vi "Periodic Tasks.vi"(8 "error in":errorcluster) -> ()   [LabVIEW 2013]
doc: "This VI runs in parallel to other tasks. It can contain as many user-defined periodic loops as you need. These can carry out PID or other sorts of timed response."
uses:
  <vilib>/Rock Robotics/WPI/Solenoid/WPI_SolenoidValue.ctl
  Drive State.ctl
  <vilib>/Rock Robotics/SystemInterfaces/Utilities/FPGA_UtilitiesLED Source.ctl
  <vilib>/Rock Robotics/SystemInterfaces/Utilities/FPGA_UtilitiesLED State.ctl
  Robot Global Data.vi
  <vilib>/Rock Robotics/WPI/Solenoid/Deprecated/WPI_SolenoidGetBool.vi
  <vilib>/Rock Robotics/WPI/Solenoid/WPI_SolenoidSetEnum.vi
  <vilib>/addons/control/pid/pid.llb/PID (DBL).vi
  <vilib>/addons/control/pid/NI_PID_pid.lvlib
panel:
  in  "Shot Time":u32
  in  "ANGLE PID":T1={"proportional gain (Kc)"=0.01, "integral time (Ti, min)"=0.0, "derivative time (Td, min)"=0.0}
  in  "Shooter Power 2":dbl=1.0
  out "Conveyor Out":dbl
  out "BM Output":dbl
  out "Arm Out":T2
  in  "Low Power":dbl=0.15
  in  "High Power":dbl=1.0
  in  "Arm Down Cov Power":dbl=0.4 format="%#_13g"
  in  "Center Power":dbl=0.2
  in  "Yaw Rate x Constant":dbl=0.1 format="%#_13g"
  in  "Rot Threshold":dbl=0.08 format="%#_13g"
  in  "FL PID":T1={"proportional gain (Kc)"=0.01, "integral time (Ti, min)"=0.1, "derivative time (Td, min)"=0.0}
  in  "FR PID":T1={"proportional gain (Kc)"=0.01, "integral time (Ti, min)"=0.1, "derivative time (Td, min)"=0.0}
  in  "BL PID":T1={"proportional gain (Kc)"=0.01, "integral time (Ti, min)"=0.1, "derivative time (Td, min)"=0.0}
  in  "BR PID":T1={"proportional gain (Kc)"=0.01, "integral time (Ti, min)"=0.1, "derivative time (Td, min)"=0.0}
  out "ANGULAR\nRATE":dbl(knob) scale=-100.0..100.0
  out "ANGLE":dbl(slide) scale=-180.0..180.0
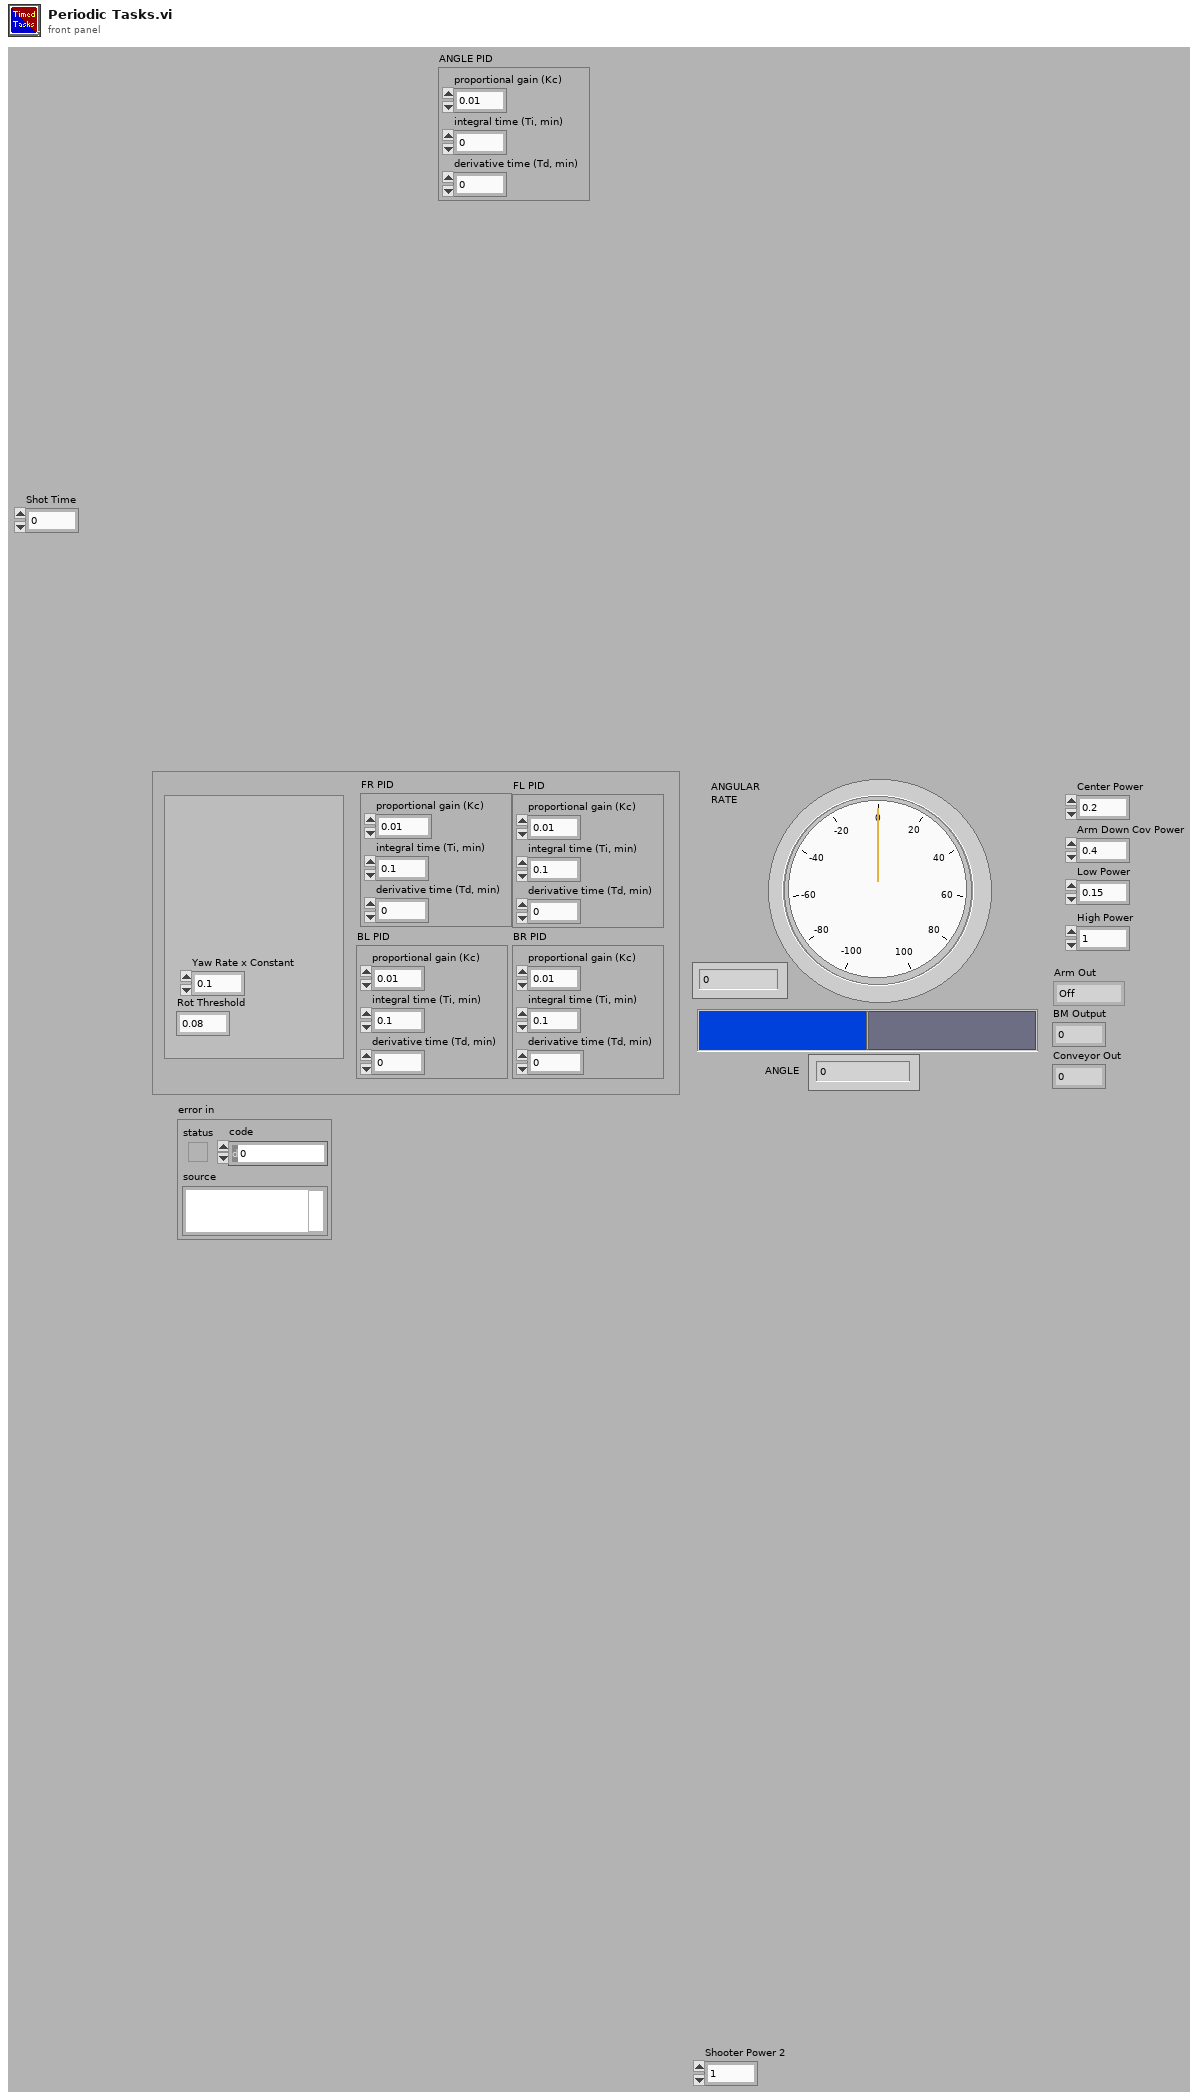
[diagram p1: front panel]
types:
  T1 = cluster{"proportional gain (Kc)":dbl, "integral time (Ti, min)":dbl, "derivative time (Td, min)":dbl}
  T2 = typedef "WPI_SolenoidValue.ctl" = enum16{"Off", "On", "Forward", "Reverse"}
  T3 = typedef "Drive State.ctl" = enum16{"Knob Control", "Straight PID", "Reset Mode"}
  T4 = typedef "WPI_MotorControlDeviceRef.ctl" = cluster{"DeviceStatus":errorcluster, "Type":enum16{"PWM", "CAN"}, "PWM":cluster{"Digital Module":T5, "PWM Channel":T6, "DeadBand":T7}, "CAN":cluster{"Device Number":u8, "Control Mode":T8, "Semaphore":T9, "Max Vout":dbl}, "Invert":bool, "TransformRef":T10, "InvTransformRef":T10}
  T5 = typedef "FPGA_TypedefDigitalModule.ctl" = enum16{"Digital Module 1", "Digital Module 2"}
  T6 = typedef "FPGA_DIOPWMChannel.ctl" = enum8{"PWM 1", "PWM 2", "PWM 3", "PWM 4", "PWM 5", "PWM 6", "PWM 7", "PWM 8", "PWM 9", "PWM 10", "Invalid"}
  T7 = typedef "WPI_PWMDeadband.ctl" = cluster{"Name":string, "maxPositivePwm":i32, "minPositivePwm":i32, "centerPwm":i32, "maxNegativePwm":i32, "minNegativePwm":i32, "angularRange":u16}
  T8 = typedef "WPI_CANJaguar_ControlMode.ctl" = enum8{"Percent VBus", "Current", "Speed", "Position", "Voltage"}
  T9 = typedef "Semaphore RefNum" = refnum<k1>
  T10 = typedef "WPI_PWMTransform_ConPane.ctl" = refnum<vi>
  T11 = typedef "WPI_EncoderDevRef.ctl" = cluster{"DevStatus":errorcluster, "EncoderIndex":T12, "CounterIndex":T13, "DistancePerCount":dbl, "Decoding Type":T14}
  T12 = typedef "FPGA_EncoderIdx.ctl" = enum8{"Enc 0", "Enc 1", "Enc 2", "Enc 3", "Invalid"}
  T13 = typedef "FPGA_CounterCtrSystemIndex.ctl" = enum8{"Ctr 0", "Ctr 1", "Ctr 2", "Ctr 3", "Ctr 4", "Ctr 5", "Ctr 6", "Ctr 7", "Invalid"}
  T14 = typedef "WPI_EncoderType.ctl" = enum16{"1x", "2x", "4x"}
  T15 = typedef "WPI_DigitalInputDevRef.ctl" = cluster{"DevStatus":errorcluster, "DIO Channel":T16, "Digital Module":T5}
  T16 = typedef "FPGA_DIOChannel.ctl" = enum8{"DIO 1", "DIO 2", "DIO 3", "DIO 4", "DIO 5", "DIO 6", "DIO 7", "DIO 8", "DIO 9", "DIO 10", "DIO 11", "DIO 12", "DIO 13", "DIO 14", "Invalid"}
  T17 = typedef "WPI_GyroDevRef.ctl" = cluster{"DevStatus":errorcluster, "Analog Module":T18, "Analog Channel":T19, "Offset":dbl, "Gain (VoltsPerDegree/Second)":dbl}
  T18 = typedef "FPGA_TypedefAnalogModule.ctl" = enum16{"Analog Module 1", "Analog Module 2"}
  T19 = typedef "FPGA_AIChannel.ctl" = enum8{"AI 1", "AI 2", "AI 3", "AI 4", "AI 5", "AI 6", "AI 7", "AI 8", "Invalid"}
  T20 = typedef "FPGA_UtilitiesLED State.ctl" = enum16{"Off", "On", "Toggle"}
  T21 = typedef "FPGA_UtilitiesLED Source.ctl" = enum16{"User LED", "FPGA LED"}
  T22 = typedef "WPI_SolenoidDevRef.ctl" = cluster{"DevStatus":errorcluster, "Solenoid Module":T23, "Forward Solenoid Channel":T24, "Reverse Solenoid Channel":T24}
  T23 = typedef "FPGA_TypedefSolenoidModule.ctl" = enum16{"Solenoid Module 1", "Solenoid Module 2"}
  T24 = typedef "WPI_SolenoidChannel.ctl" = enum8{"Solenoid 1", "Solenoid 2", "Solenoid 3", "Solenoid 4", "Solenoid 5", "Solenoid 6", "Solenoid 7", "Solenoid 8", "Invalid"}
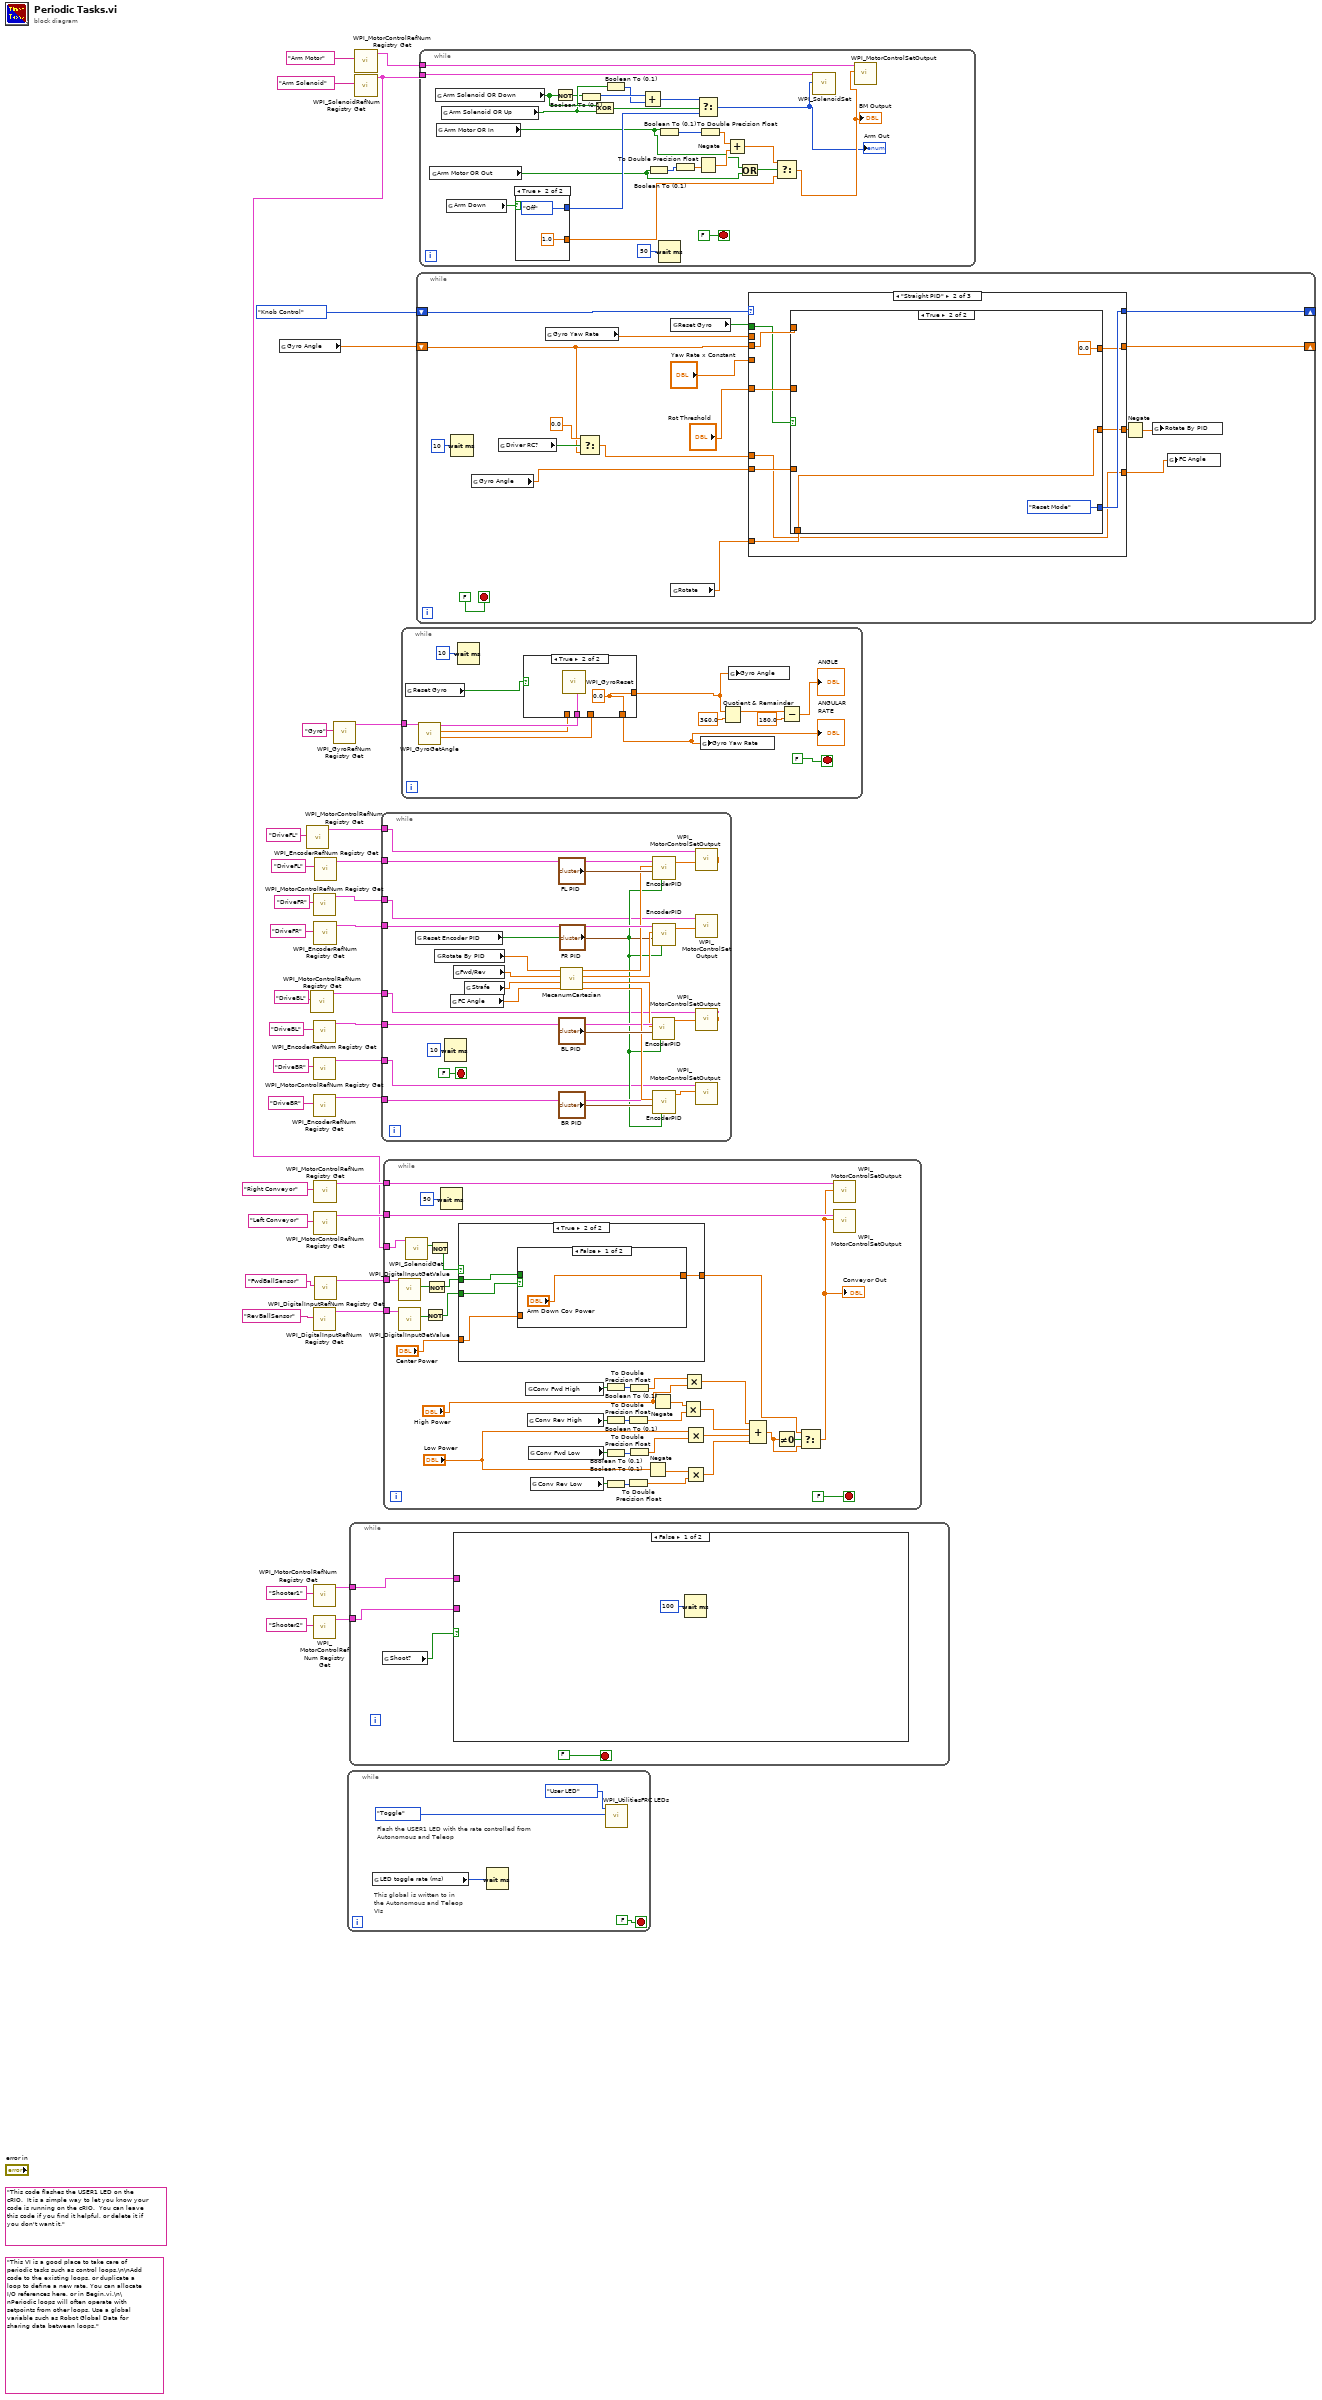
[diagram p0: block diagram]
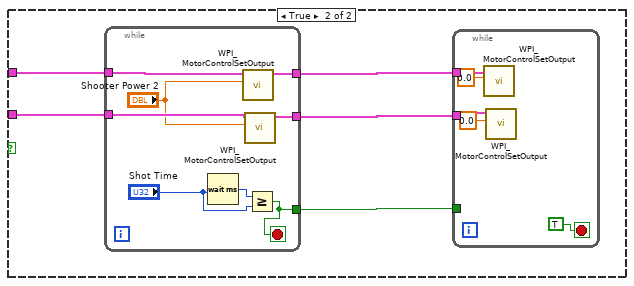
[diagram p2: hidden frame]
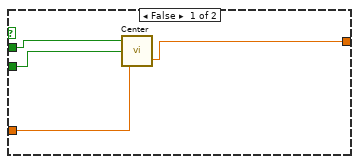
[diagram p3: hidden frame]
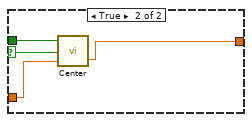
[diagram p4: hidden frame]
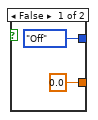
[diagram p5: hidden frame]
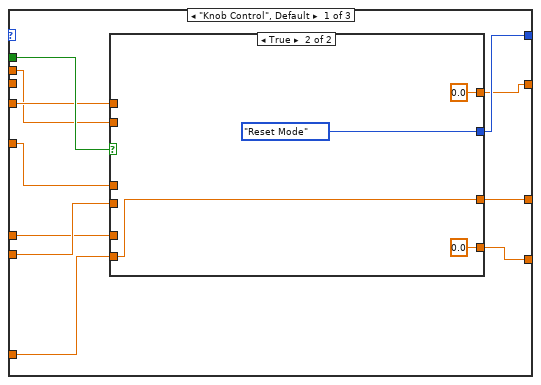
[diagram p6: hidden frame]
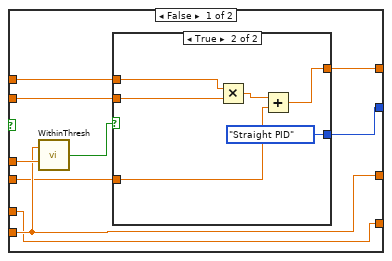
[diagram p7: hidden frame]
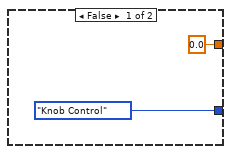
[diagram p8: hidden frame]
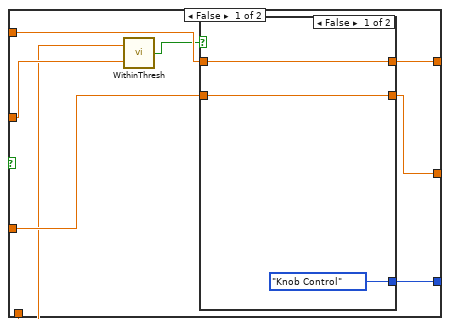
[diagram p9: hidden frame]
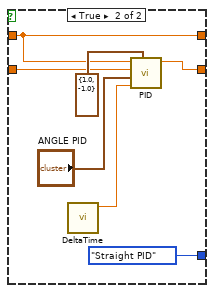
[diagram p10: hidden frame]
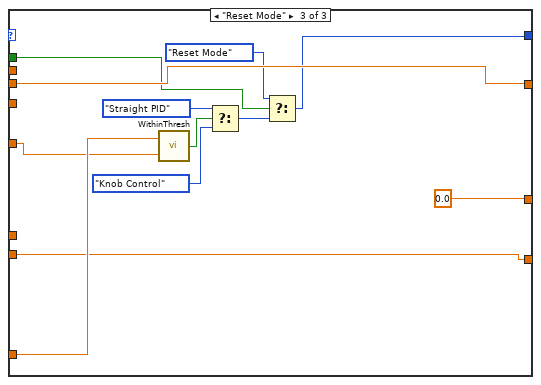
[diagram p11: hidden frame]
diagram:
  (unwired) "This code flashes the USER1 LED on the cRIO.  It is a simple way to let you know your code is running on the cRIO.  You can leave this code if you find it helpful, or delete it if you don't want it."
  (unwired) "This VI is a good place to take care of periodic tasks such as control loops.\n\nAdd code to the existing loops, or duplicate a loop to define a new rate. You can allocate I/O references here, or in Begin.vi.\n\nPeriodic loops will often operate with setpoints from other loops. Use a global variable such as Robot Global Data for sharing data between loops."
  n1 = global read "Robot Global Data.vi" "Gyro Angle"() -> (w6:dbl)
  n2 = call <vilib>:"WPI_MotorControlRefNum Registry Get.vi"("refnum name"="DriveFL") -> ("MotorControlDevRef"=w15:T4)  [unwired: 9 in, 1 out]
  n3 = call <vilib>:"WPI_MotorControlRefNum Registry Get.vi"("refnum name"="DriveBL") -> ("MotorControlDevRef"=w19:T4)  [unwired: 9 in, 1 out]
  n4 = call <vilib>:"WPI_MotorControlRefNum Registry Get.vi"("refnum name"="DriveFR") -> ("MotorControlDevRef"=w17:T4)  [unwired: 9 in, 1 out]
  n5 = call <vilib>:"WPI_EncoderRefNum Registry Get.vi"("refnum name"="DriveBL") -> ("EncoderDevRef"=w36:T11)  [unwired: 9 in, 1 out]
  n6 = call <vilib>:"WPI_MotorControlRefNum Registry Get.vi"("refnum name"="DriveBR") -> ("MotorControlDevRef"=w21:T4)  [unwired: 9 in, 1 out]
  n7 = call <vilib>:"WPI_EncoderRefNum Registry Get.vi"("refnum name"="DriveBR") -> ("EncoderDevRef"=w34:T11)  [unwired: 9 in, 1 out]
  n8 = call <vilib>:"WPI_DigitalInputRefNum Registry Get.vi"("refnum name"="RevBallSensor") -> ("DigitalInputDevRef"=w7:T15)  [unwired: 9 in, 1 out]
  n9 = call <vilib>:"WPI_MotorControlRefNum Registry Get.vi"("refnum name"="Shooter1") -> ("MotorControlDevRef"=w3:T4)  [unwired: 9 in, 1 out]
  n10 = call <vilib>:"WPI_MotorControlRefNum Registry Get.vi"("refnum name"="Shooter2") -> ("MotorControlDevRef"=w2:T4)  [unwired: 9 in, 1 out]
  n11 = call <vilib>:"WPI_EncoderRefNum Registry Get.vi"("refnum name"="DriveFR") -> ("EncoderDevRef"=w35:T11)  [unwired: 9 in, 1 out]
  n12 = call <vilib>:"WPI_MotorControlRefNum Registry Get.vi"("refnum name"="Right Conveyor") -> ("MotorControlDevRef"=w12:T4)  [unwired: 9 in, 1 out]
  n13 = call <vilib>:"WPI_MotorControlRefNum Registry Get.vi"("refnum name"="Left Conveyor") -> ("MotorControlDevRef"=w11:T4)  [unwired: 9 in, 1 out]
  n14 = call <vilib>:"WPI_EncoderRefNum Registry Get.vi"("refnum name"="DriveFL") -> ("EncoderDevRef"=w28:T11)  [unwired: 9 in, 1 out]
  n15 = call <vilib>:"WPI_DigitalInputRefNum Registry Get.vi"("refnum name"="FwdBallSensor") -> ("DigitalInputDevRef"=w8:T15)  [unwired: 9 in, 1 out]
  n16 = call <vilib>:"WPI_GyroRefNum Registry Get.vi"("refnum name"="Gyro") -> ("GyroDevRef"=w24:T17)  [unwired: 9 in, 1 out]
  n17 = while {
    stop <- FALSE stop-if-true
    # "This global is written to in the Autonomous and Teleop VIs"
    # "Flash the USER1 LED with the rate controlled from Autonomous and Teleop"
    n18 = global read "Robot Global Data.vi" "LED toggle rate (ms)"() -> (w37:u32)
    n19 = Wait (ms)(milliseconds to wait=w37) -> ()  [unwired: 1 out]
    n20 = call <vilib>:"WPI_UtilitiesFRC LEDs.vi"("State"=FPGA_UtilitiesLED_State."Toggle", "LED Type"=FPGA_UtilitiesLED_Source."User LED") -> ()  [unwired: 1 in, 9 out]
  }
  n21 = while {
    tunnel: w3 -> [w42]
    tunnel: w2 -> [w43]
    stop <- FALSE stop-if-true
    n22 = global read "Robot Global Data.vi" "Shoot?"() -> (w41:bool)
    n23 = case shown="False" w41 {
      tunnel: w43 -> [_ w50]
      tunnel: w42 -> [_ w49]
      frame False {
        n24 = Wait (ms)(milliseconds to wait=u32 100) -> ()  [unwired: 1 out]
      }
      frame True {
        n25 = while {
          tunnel: w50 -> [w63]
          tunnel: w49 -> [w62]
          tunnel: [w58] -> w48
          tunnel: [w57] -> w47
          tunnel: [w56] -> w46
          stop <- w58 stop-if-true
          n26 = Wait (ms)(milliseconds to wait="Shot Time") -> (millisecond timer value=w60:u32)
          n27 = call <vilib>:"WPI_MotorControlSetOutput.vi"("Output"="Shooter Power 2", "MotorControlDevRef"=w62) -> ("MotorControlDevRef"=w57:T4)  [unwired: 7 in, 2 out]
          n28 = call <vilib>:"WPI_MotorControlSetOutput.vi"("Output"="Shooter Power 2", "MotorControlDevRef"=w63) -> ("MotorControlDevRef"=w56:T4)  [unwired: 7 in, 2 out]
          n29 = Greater Or Equal?(x=w60, y="Shot Time") -> (x >= y?=w58:bool)
        }
        n30 = while {
          tunnel: w48 -> [_]
          tunnel: w47 -> [w54]
          tunnel: w46 -> [w55]
          stop <- TRUE stop-if-true
          n31 = call <vilib>:"WPI_MotorControlSetOutput.vi"("Output"=0.0, "MotorControlDevRef"=w54) -> ()  [unwired: 7 in, 3 out]
          n32 = call <vilib>:"WPI_MotorControlSetOutput.vi"("Output"=0.0, "MotorControlDevRef"=w55) -> ()  [unwired: 7 in, 3 out]
        }
      }
    }
  }
  n33 = call <vilib>:"WPI_MotorControlRefNum Registry Get.vi"("refnum name"="Arm Motor") -> ("MotorControlDevRef"=w27:T4)  [unwired: 9 in, 1 out]
  n34 = call <vilib>:"WPI_SolenoidRefNum Registry Get.vi"("refnum name"="Arm Solenoid") -> ("SolenoidDevRef"=w1:T22)  [unwired: 9 in, 1 out]
  n35 = while {
    tunnel: w36 -> [w75]
    tunnel: w35 -> [w79]
    tunnel: w28 -> [w70]
    tunnel: w34 -> [w74]
    tunnel: w21 -> [w68]
    tunnel: w19 -> [w67]
    tunnel: w17 -> [w66]
    tunnel: w15 -> [w65]
    stop <- FALSE stop-if-true
    n36 = global read "Robot Global Data.vi" "Reset Encoder PID"() -> (w71:bool)
    n37 = global read "Robot Global Data.vi" "Rotate By PID"() -> (w69:dbl)
    n38 = Wait (ms)(milliseconds to wait=u32 10) -> ()  [unwired: 1 out]
    n39 = global read "Robot Global Data.vi" "FC Angle"() -> (w64:dbl)
    n40 = global read "Robot Global Data.vi" "Fwd/Rev"() -> (w88:dbl)
    n41 = global read "Robot Global Data.vi" "Strafe"() -> (w87:dbl)
    n42 = call "MecanumCartesian.vi"("Gyro Angle"=w64, "X"=w87, "Y"=w88, "Rotation"=w69) -> ("Rear Right"=w76:dbl, "Rear Left"=w73:dbl, "Front Right"=w77:dbl, "Front Left"=w78:dbl)
    n43 = call "EncoderPID.vi"("Reset"=w71, "PID gains"="BL PID", "Wheel"=w73, "EncoderRef"=w75) -> ("output"=w82:dbl)  [unwired: 3 in, 2 out]
    n44 = call "EncoderPID.vi"("Reset"=w71, "PID gains"="FL PID", "Wheel"=w78, "EncoderRef"=w70) -> ("output"=w81:dbl)  [unwired: 3 in, 2 out]
    n45 = call "EncoderPID.vi"("Reset"=w71, "PID gains"="FR PID", "Wheel"=w77, "EncoderRef"=w79) -> ("output"=w83:dbl)  [unwired: 3 in, 2 out]
    n46 = call "EncoderPID.vi"("Reset"=w71, "PID gains"="BR PID", "Wheel"=w76, "EncoderRef"=w74) -> ("output"=w80:dbl)  [unwired: 3 in, 2 out]
    n47 = call <vilib>:"WPI_MotorControlSetOutput.vi"("Output"=w81, "MotorControlDevRef"=w65) -> ()  [unwired: 7 in, 3 out]
    n48 = call <vilib>:"WPI_MotorControlSetOutput.vi"("Output"=w83, "MotorControlDevRef"=w66) -> ()  [unwired: 7 in, 3 out]
    n49 = call <vilib>:"WPI_MotorControlSetOutput.vi"("Output"=w82, "MotorControlDevRef"=w67) -> ()  [unwired: 7 in, 3 out]
    n50 = call <vilib>:"WPI_MotorControlSetOutput.vi"("Output"=w80, "MotorControlDevRef"=w68) -> ()  [unwired: 7 in, 3 out]
  }
  n51 = while {
    tunnel: w12 -> [w126]
    tunnel: w11 -> [w125]
    tunnel: w1 -> [w124]
    tunnel: w8 -> [w122]
    tunnel: w7 -> [w121]
    stop <- FALSE stop-if-true
    n52 = call <vilib>:"WPI_DigitalInputGetValue.vi"("DigitalInputDevRef"=w122) -> ("Value"=w119:bool)  [unwired: 8 in, 2 out]
    n53 = call <vilib>:"WPI_DigitalInputGetValue.vi"("DigitalInputDevRef"=w121) -> ("Value"=w120:bool)  [unwired: 8 in, 2 out]
    n54 = call-poly <vilib>:"WPI_SolenoidGet.vi"("SolenoidDevRef"=w124) -> ("Value"=w123:bool)  [unwired: 8 in, 2 out]
    n55 = Not(x=w120) -> (.not. x?=w118:bool)
    n56 = Not(x=w119) -> (.not. x?=w117:bool)
    n57 = Not(x=w123) -> (.not. x?=w115:bool)
    n58 = Wait (ms)(milliseconds to wait=u32 50) -> ()  [unwired: 1 out]
    n59 = case shown="True" w115 {
      tunnel: w118 -> [w131 w136]
      tunnel: [w129 w135] -> w94
      tunnel: w117 -> [w132 w134]
      tunnel: "Center Power" -> [w130 w133]
      frame False {
        n60 = call "Center.vi"("Power"=w130, "Rev"=w131, "Fwd"=w132) -> ("Center Power"=w129:dbl)  [unwired: 1 out]
      }
      frame True {
        n61 = case shown="False" w136 {
          selector: w136 -> [_ w139]
          tunnel: ["Arm Down Cov Power" w141] -> w135
          tunnel: w134 -> [_ w140]
          tunnel: w133 -> [_ w138]
          frame False {
          }
          frame True {
            n62 = call "Center.vi"("Power"=w138, "Rev"=w139, "Fwd"=w140) -> ("Center Power"=w141:dbl)  [unwired: 1 out]
          }
        }
      }
    }
    n63 = global read "Robot Global Data.vi" "Conv Fwd High"() -> (w114:bool)
    n64 = global read "Robot Global Data.vi" "Conv Rev High"() -> (w113:bool)
    n65 = global read "Robot Global Data.vi" "Conv Fwd Low"() -> (w111:bool)
    n66 = global read "Robot Global Data.vi" "Conv Rev Low"() -> (w112:bool)
    n67 = Boolean To (0,1)(Boolean=w114) -> (0, 1=w110:i16)
    n68 = Boolean To (0,1)(Boolean=w113) -> (0, 1=w108:i16)
    n69 = Boolean To (0,1)(Boolean=w111) -> (0, 1=w109:i16)
    n70 = Boolean To (0,1)(Boolean=w112) -> (0, 1=w92:i16)
    n71 = To Double Precision Float(number=w108) -> (double precision float=w100:dbl)
    n72 = To Double Precision Float(number=w92) -> (double precision float=w91:dbl)
    n73 = To Double Precision Float(number=w110) -> (double precision float=w107:dbl)
    n74 = To Double Precision Float(number=w109) -> (double precision float=w98:dbl)
    n75 = Negate(x="Low Power") -> (-x=w101:dbl)
    n76 = Negate(x="High Power") -> (-x=w99:dbl)
    n77 = Multiply(x=w99, y=w100) -> (x*y=w104:dbl)
    n78 = Multiply(x=w107, y="High Power") -> (x*y=w103:dbl)
    n79 = Multiply(x="Low Power", y=w98) -> (x*y=w105:dbl)
    n80 = Multiply(x=w101, y=w91) -> (x*y=w106:dbl)
    n81 = Compound Arithmetic op=ADD(w103, w104, w105, w106) -> (w97:dbl)
    n82 = Not Equal To 0?(x=w97) -> (x != 0?=w102:bool)
    n83 = Select(t=w94, s=w102, f=w97) -> (s? t:f=w93:dbl)
    "Conveyor Out" <- w93
    n84 = call <vilib>:"WPI_MotorControlSetOutput.vi"("Output"=w93, "MotorControlDevRef"=w126) -> ()  [unwired: 7 in, 3 out]
    n85 = call <vilib>:"WPI_MotorControlSetOutput.vi"("Output"=w93, "MotorControlDevRef"=w125) -> ()  [unwired: 7 in, 3 out]
  }
  n86 = while {
    tunnel: w24 -> [w148]
    stop <- FALSE stop-if-true
    n87 = global read "Robot Global Data.vi" "Reset Gyro"() -> (w147:bool)
    n88 = call <vilib>:"WPI_GyroGetAngle.vi"("GyroDevRef"=w148) -> ("Angular Rate"=w142:dbl, "Angle"=w143:dbl, "GyroDevRef"=w146:T17)  [unwired: 7 in, 1 out]
    n89 = Wait (ms)(milliseconds to wait=u32 10) -> ()  [unwired: 1 out]
    n90 = case shown="True" w147 {
      tunnel: w146 -> [_ w158]
      tunnel: [w156 w157] -> w145
      tunnel: [w155 w157] -> w144
      tunnel: w143 -> [w156 _]
      tunnel: w142 -> [w155 _]
      frame False {
      }
      frame True {
        w157 = 0.0
        n91 = call <vilib>:"WPI_GyroReset.vi"("GyroDevRef"=w158) -> ()  [unwired: 9 in, 2 out]
      }
    }
    "ANGULAR\nRATE" <- w144
    n92 = global write "Robot Global Data.vi" "Gyro Yaw Rate"(w144) -> ()
    n93 = Quotient & Remainder(x=w145, y=360.0) -> (x-y*floor(x/y)=w151:dbl)  [unwired: 1 out]
    n94 = global write "Robot Global Data.vi" "Gyro Angle"(w145) -> ()
    n95 = Subtract(x=w151, y=180.0) -> (x-y=→"ANGLE":dbl)
  }
  n96 = while {
    shift-right: [w174] -> _
    shift-left: w6 -> [w159]
    shift-right: [w175] -> _
    shift-left: Drive_State."Knob Control" ("Drive State") -> [w173]
    stop <- FALSE stop-if-true
    n97 = Wait (ms)(milliseconds to wait=u32 10) -> ()  [unwired: 1 out]
    n98 = global read "Robot Global Data.vi" "Gyro Angle"() -> (w164:dbl)
    n99 = global read "Robot Global Data.vi" "Driver RC?"() -> (w165:bool)
    n100 = global read "Robot Global Data.vi" "Gyro Yaw Rate"() -> (w172:dbl)
    n101 = Select(t=0.0, s=w165, f=w159) -> (s? t:f=w162:dbl)
    n102 = global read "Robot Global Data.vi" "Reset Gyro"() -> (w161:bool)
    n103 = global read "Robot Global Data.vi" "Rotate"() -> (w168:dbl)
    n104 = case shown="\"Straight PID\"" w173 {
      tunnel: "Rot Threshold" -> [w183 w214 w242]
      tunnel: [w186 w217 w248] -> w175
      tunnel: w172 -> [w180 _ _]
      tunnel: "Yaw Rate x Constant" -> [w181 _ _]
      tunnel: [w182 w216 w250] -> w174
      tunnel: w159 -> [_ w215 w250]
      tunnel: w164 -> [w179 w213 w239]
      tunnel: w168 -> [w184 w211 w243]
      tunnel: [w185 w212 0.0 ("output")] -> w167
      tunnel: w162 -> [w177 w210 _]
      tunnel: w161 -> [w187 w209 w240]
      tunnel: [w178 w210 w239] -> w160
      frame "Knob Control", Default {
        n105 = case shown="True" w187 {
          tunnel: [w188 Drive_State."Reset Mode" ("Drive State")] -> w186
          tunnel: [w193 w207] -> w185
          tunnel: w184 -> [w193 w207]
          tunnel: w183 -> [w196 _]
          tunnel: [w194 0.0] -> w182
          tunnel: w181 -> [w192 _]
          tunnel: w180 -> [w191 _]
          tunnel: w179 -> [w190 _]
          tunnel: [w189 0.0 ("Gyro Angle")] -> w178
          tunnel: w177 -> [w189 _]
          frame False {
            n106 = call "WithinThresh.vi"("Threshold"=w196, "In"=w193) -> ("Within Thresh?"=w195:bool)
            n107 = case shown="True" w195 {
              tunnel: [0.0 w204] -> w194
              tunnel: w192 -> [_ w202]
              tunnel: w191 -> [_ w201]
              tunnel: w190 -> [_ w200]
              tunnel: [Drive_State."Knob Control" ("Drive State") Drive_State."Straight PID" ("Drive State")] -> w188
              frame False {
              }
              frame True {
                n108 = Multiply(x=w202, y=w201) -> (x*y=w203:dbl)
                n109 = Add(x=w203, y=w200) -> (x+y=w204:dbl)
              }
            }
          }
          frame True {
          }
        }
      }
      frame "Straight PID" {
        n110 = case shown="True" w209 {
          tunnel: [w225 Drive_State."Reset Mode" ("Drive State")] -> w217
          tunnel: [w224 0.0 ("Gyro Angle")] -> w216
          tunnel: w215 -> [w223 _]
          tunnel: w214 -> [w221 _]
          tunnel: w213 -> [w220 _]
          tunnel: [w219 w237] -> w212
          tunnel: w211 -> [w218 w237]
          frame False {
            n111 = call "WithinThresh.vi"("Threshold"=w221, "In"=w218) -> ("Within Thresh?"=w222:bool)
            n112 = case shown="False" w222 {
              tunnel: [Drive_State."Knob Control" ("Drive State") Drive_State."Straight PID" ("Drive State")] -> w225
              tunnel: [w226 w229] -> w224
              tunnel: w223 -> [w226 w229]
              tunnel: w220 -> [w228 w231]
              tunnel: [w228 w230] -> w219
              frame False {
              }
              frame True {
                n113 = call "DeltaTime.vi"() -> ("dt"=w233:dbl)  [unwired: 11 in]
                n114 = call-poly <vilib>:"PID.vi"("output range"=cluster{"output high":dbl, "output low":dbl} {"output high"=1.0, "output low"=-1.0}, "dt (s)"=w233, "PID gains"="ANGLE PID", "process variable"=w231, "setpoint"=w229) -> ("output"=w230:dbl)  [unwired: 5 in, 1 out]
              }
            }
          }
          frame True {
          }
        }
      }
      frame "Reset Mode" {
        n115 = call "WithinThresh.vi"("Threshold"=w242, "In"=w243) -> ("Within Thresh?"=w246:bool)
        n116 = Select(t=Drive_State."Straight PID" ("Drive State"), s=w246, f=Drive_State."Knob Control" ("Drive State")) -> (s? t:f=w247:T3)
        n117 = Select(t=Drive_State."Reset Mode" ("Drive State"), s=w240, f=w247) -> (s? t:f=w248:T3)
      }
    }
    n118 = Negate(x=w167) -> (-x=w166:dbl)
    n119 = global write "Robot Global Data.vi" "Rotate By PID"(w166) -> ()
    n120 = global write "Robot Global Data.vi" "FC Angle"(w160) -> ()
  }
  n121 = while {
    tunnel: w27 -> [w272]
    tunnel: w1 -> [w271]
    stop <- FALSE stop-if-true
    n122 = global read "Robot Global Data.vi" "Arm Motor OR Out"() -> (w255:bool)
    n123 = global read "Robot Global Data.vi" "Arm Solenoid OR Down"() -> (w268:bool)
    n124 = global read "Robot Global Data.vi" "Arm Motor OR In"() -> (w256:bool)
    n125 = global read "Robot Global Data.vi" "Arm Solenoid OR Up"() -> (w264:bool)
    n126 = global read "Robot Global Data.vi" "Arm Down"() -> (w273:bool)
    n127 = case shown="True" w273 {
      tunnel: [0.0 ("Output") 1.0 ("Output")] -> w253
      tunnel: [WPI_SolenoidValue."Off" ("Value") WPI_SolenoidValue."Off" ("Value")] -> w269
      frame False {
      }
      frame True {
      }
    }
    n128 = Not(x=w268) -> (.not. x?=w263:bool)
    n129 = Boolean To (0,1)(Boolean=w263) -> (0, 1=w267:i16)
    n130 = Exclusive Or(1:w264, 2:w268) -> (0:w270:bool)
    n131 = Boolean To (0,1)(Boolean=w264) -> (0, 1=w266:i16)
    n132 = Add(x=w267, y=w266) -> (x+y=w265:i16)
    n133 = Boolean To (0,1)(Boolean=w255) -> (0, 1=w260:i16)
    n134 = Boolean To (0,1)(Boolean=w256) -> (0, 1=w261:i16)
    n135 = Wait (ms)(milliseconds to wait=u32 50) -> ()  [unwired: 1 out]
    n136 = To Double Precision Float(number=w260) -> (double precision float=w259:dbl)
    n137 = Select(t=w265, s=w270, f=w269) -> (s? t:f=w251:u16)
    "Arm Out" <- w251
    n138 = Negate(x=w259) -> (-x=w258:dbl)
    n139 = To Double Precision Float(number=w261) -> (double precision float=w262:dbl)
    n140 = Add(x=w262, y=w258) -> (x+y=w254:dbl)
    n141 = Or(x=w256, y=w255) -> (x .or. y?=w257:bool)
    n142 = Select(t=w254, s=w257, f=w253) -> (s? t:f=w252:dbl)
    "BM Output" <- w252
    n143 = call-poly <vilib>:"WPI_SolenoidSet.vi"("Value"=w251, "SolenoidDevRef"=w271) -> ()  [unwired: 8 in, 2 out]
    n144 = call <vilib>:"WPI_MotorControlSetOutput.vi"("Output"=w252, "MotorControlDevRef"=w272) -> ()  [unwired: 7 in, 3 out]
  }
